vi "KB-Result show.vi"(10 "CCD Hand Array":refnum<vi>[](array[refnum]), 11 "Data Result":string[][](table)) -> ()   [LabVIEW 2015]
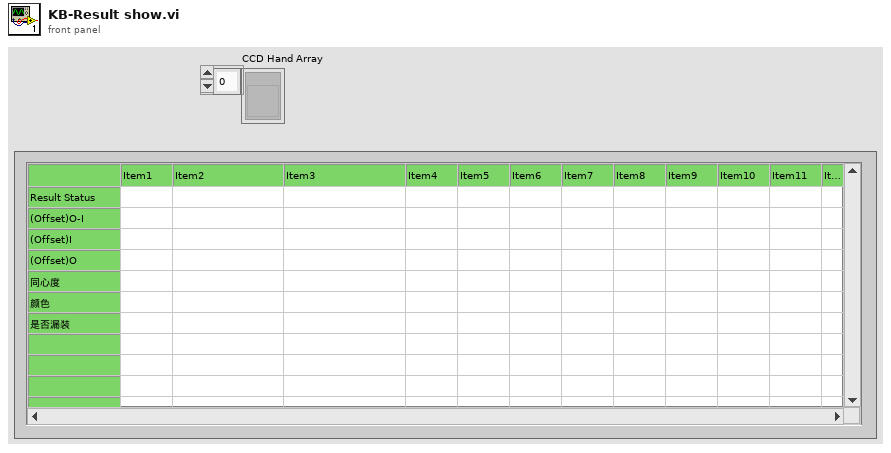
[diagram p1: front panel]
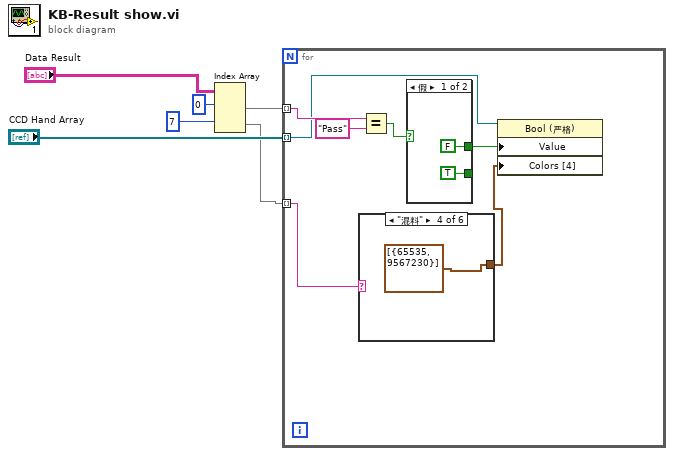
[diagram p0: block diagram]
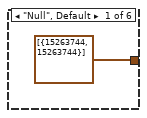
[diagram p2: hidden frame]
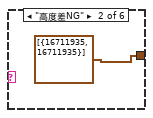
[diagram p3: hidden frame]
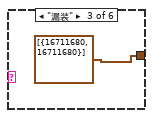
[diagram p4: hidden frame]
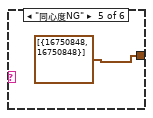
[diagram p5: hidden frame]
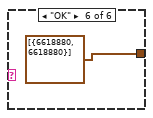
[diagram p6: hidden frame]
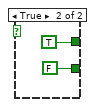
[diagram p7: hidden frame]
diagram:
  n1 = Index Array(array="Data Result", index (row) #1=0 ("索引 (行)"), index (row) #2=7 ("索引 (行)")) -> (element #1=w4:string[], element #2=w1:string[])  [unwired: 2 in]
  n2 = for {
    tunnel: w4 -> [w13] mode=indexing
    tunnel: "CCD Hand Array" -> [w12] mode=indexing
    tunnel: w1 -> [w8] mode=indexing
    n3 = case shown="\"混料\"" w8 {
      tunnel: [cluster{u32, u32}[] [{15263744, 15263744}] ("颜色[4]") cluster{u32, u32}[] [{16711935, 16711935}] ("颜色[4]") cluster{u32, u32}[] [{16711680, 16711680}] ("颜色[4]") cluster{u32, u32}[] [{65535, 9567230}] ("颜色[4]") cluster{u32, u32}[] [{16750848, 16750848}] ("颜色[4]") cluster{u32, u32}[] [{6618880, 6618880}] ("颜色[4]")] -> w7
      frame "Null", Default {
      }
      frame "高度差NG" {
      }
      frame "漏装" {
      }
      frame "混料" {
      }
      frame "同心度NG" {
      }
      frame "OK" {
      }
    }
    n4 = Equal?(x=w13, y="Pass") -> (x = y?=w10:bool)
    n5 = case shown="假" w10 {
      tunnel: [FALSE TRUE] -> w9
      tunnel: [TRUE FALSE] -> _
      frame False {
      }
      frame True {
      }
    }
    n6 = property class="Bool (严格)"(reference=w12, "Value"=w9, "Colors [4]"=w7) -> ()  [unwired: 1 in, 2 out]
  }
